vi "Inheritance Example Subvi.vi"(1 "Array":refnum<class "Packet.lvclass">[](array[class])) -> (0 "Array 2":T1[](array[typedef]))   [LabVIEW 2019]
uses:
  Code/Shared/TCP Packet/Packet.lvclass
  Code/Shared/TCP Packet/packet type STYP.ctl
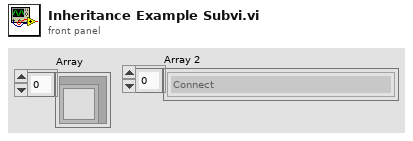
[diagram p1: front panel]
types:
  T1 = typedef "Packet.lvclass/packet type STYP.ctl" = enum16{"Connect", "Disconnect", "Direction", "Score", "Map"}
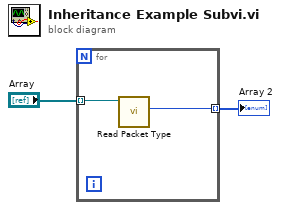
[diagram p0: block diagram]
diagram:
  n1 = for {
    tunnel: "Array" -> [w4] mode=indexing
    tunnel: [w3] -> w1 mode=indexing
    n2 = call-dynamic "Read Packet Type.vi"("Packet in"=w4) -> ("Enum"=w3:T1)  [unwired: 8 in, 2 out]
  }
  "Array 2" <- w1
